vi "GetUnwiredOutputs.vi"(11 "SubVIs":refnum<vi>[](array[refnum])) -> (0 "error out":errorcluster, 3 "Terminals[]":refnum<vi>[](array[refnum]))   [LabVIEW 2016]
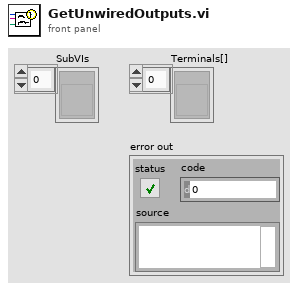
[diagram p1: front panel]
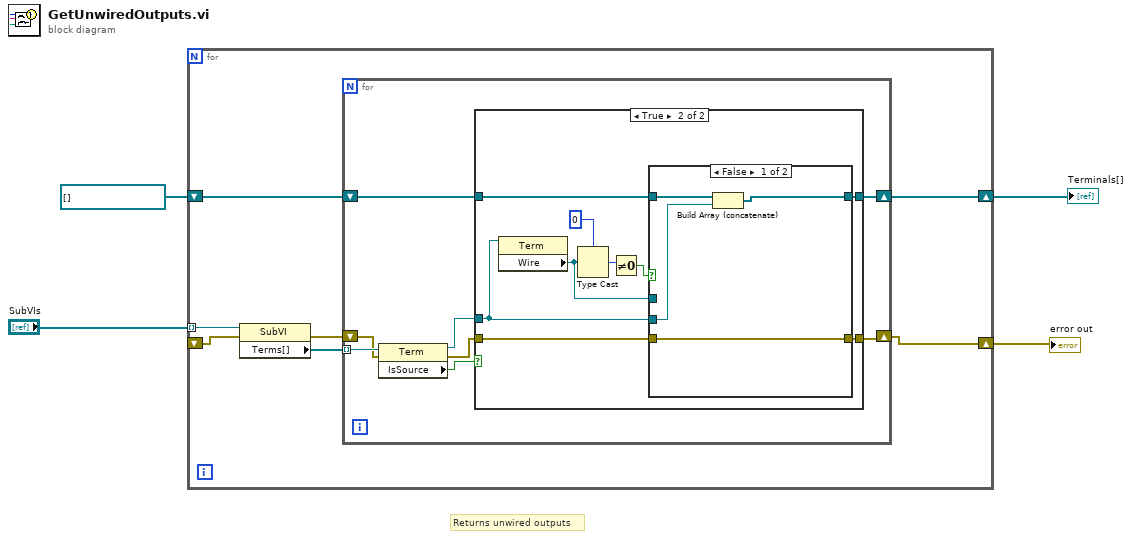
[diagram p0: block diagram]
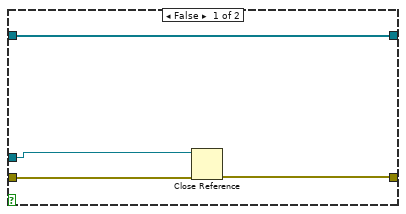
[diagram p2: hidden frame]
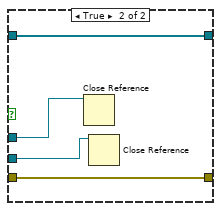
[diagram p3: hidden frame]
diagram:
  # "Returns unwired outputs"
  n1 = for {
    tunnel: "SubVIs" -> [w10] mode=indexing
    shift-right: [w8] -> w4
    shift-left: refnum<vi>[] [] ("Terminals[]") -> [w9]
    shift-right: [w6] -> w3
    shift-left: _ -> [w5]
    n2 = property class="SubVI"(reference=w10, error in=w5) -> (error out=w7:errorcluster, "Terms[]"=w11:refnum<vi>[])  [unwired: 1 out]
    n3 = for {
      tunnel: w11 -> [w19] mode=indexing
      shift-right: [w15] -> w8
      shift-left: w9 -> [w16]
      shift-right: [w12] -> w6
      shift-left: w7 -> [w13]
      n4 = property class="Term"(reference=w19, error in=w13) -> (reference out=w17:refnum<vi>, error out=w14:errorcluster, "IsSource"=w18:bool)
      n5 = case shown="True" w18 {
        tunnel: w17 -> [w22 w29]
        tunnel: w16 -> [w23 w32]
        tunnel: [w23 w31] -> w15
        tunnel: w14 -> [w21 w30]
        tunnel: [w20 w24] -> w12
        frame False {
          n6 = Close Reference(reference=w22, error in (no error)=w21) -> (error out=w20:errorcluster)
        }
        frame True {
          n7 = property class="Term"(reference=w29) -> ("Wire"=w25:refnum<vi>)  [unwired: 1 in, 2 out]
          n8 = Type Cast(type=0, x=w25) -> (*(type *) &x=w26:i32)
          n9 = Not Equal To 0?(x=w26) -> (x != 0?=w28:bool)
          n10 = case shown="False" w28 {
            tunnel: w32 -> [w36 w39]
            tunnel: [w35 w39] -> w31
            tunnel: w30 -> [w33 w37]
            tunnel: w29 -> [w34 w40]
            tunnel: w25 -> [_ w38]
            tunnel: [w33 w37] -> w24
            frame False {
              n11 = Build Array (concatenate)(w36, w34) -> (w35:refnum<vi>[])
            }
            frame True {
              n12 = Close Reference(reference=w38) -> ()  [unwired: 1 in, 1 out]
              n13 = Close Reference(reference=w40) -> ()  [unwired: 1 in, 1 out]
            }
          }
        }
      }
    }
  }
  "Terminals[]" <- w4
  "error out" <- w3
